vi "FCI_EON_Blob_Center.vi"(8 "error in (no error)":errorcluster, 10 "Coord ROI":T1 {"Contours"."Type" items=["No Selection", "Point", "Line", "Rectangle", "Oval", "Polygon", "Freehand Region", "Annulus", "Unused2", "Unused3", "Broken Line", "Freehand Line", "Rotated Rectangle"]}, 11 "Image In":T2(plugin-control)) -> (0 "error out":errorcluster, 1 "EON Area":dbl, 2 "EON Presence/Absence":bool, 3 "Blob Center":cluster{"Center X":dbl, "Center Y":dbl})   [LabVIEW 2019, in "Algorithm.lvclass"]
uses:
  FrameworkOverrides/Algorithm.lvclass
  <vilib>/vision/NI_Vision_Development_Module.lvlib
panel:
  out "Y Coord":dbl[](array[numeric])
  out "Number of Particles":i32
  out "subarray 2":dbl[](array[numeric])
  out "index of element":i32
  out "Array":bool[](array[boolean])
  out "X Coord":dbl[](array[numeric])
  out "Image 2":T2(plugin-control)
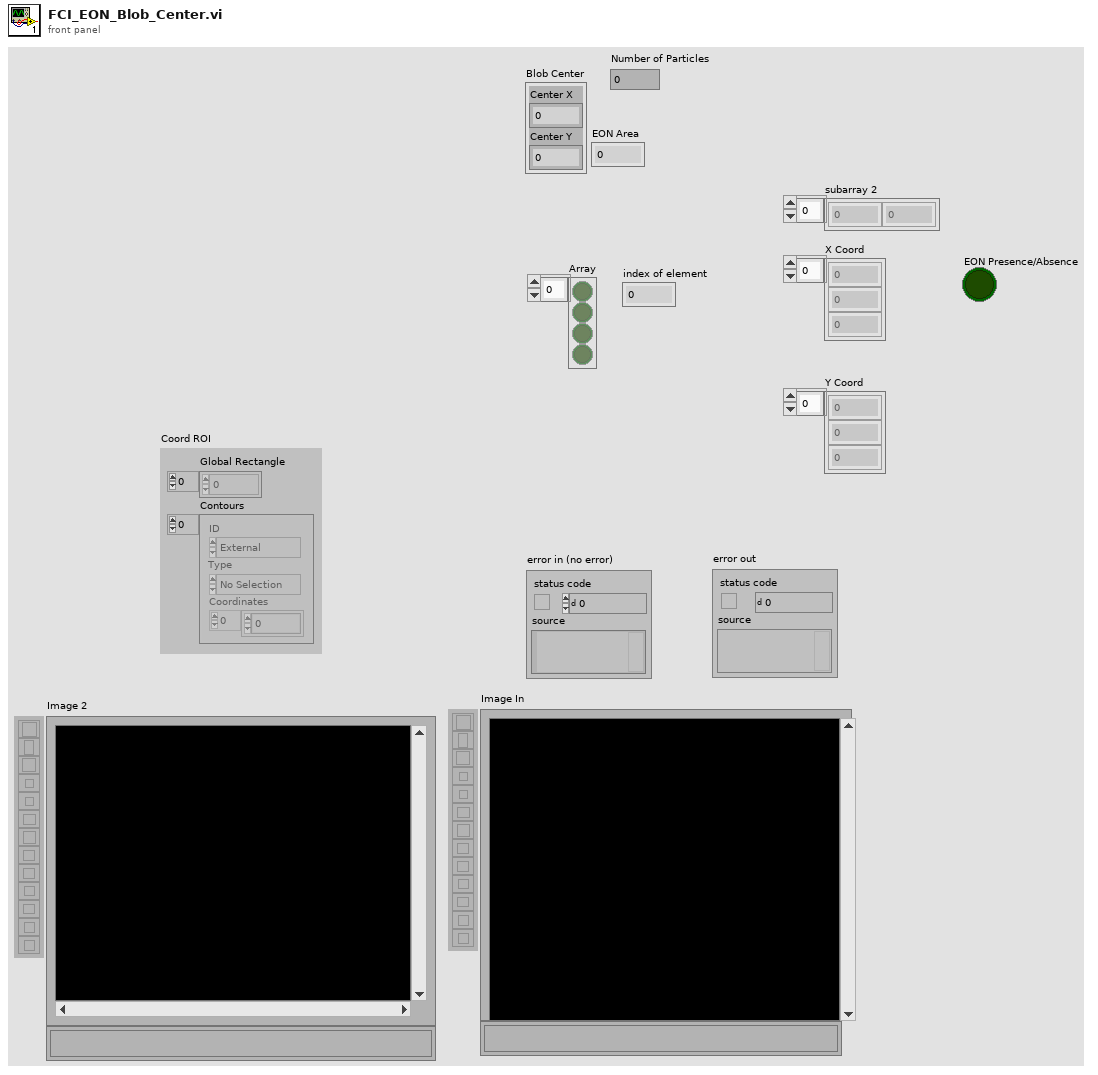
[diagram p1: front panel]
types:
  T1 = typedef "ROI Descriptor" = cluster{"Global Rectangle":i32[], "Contours":cluster{"ID":enum32{"External", "Internal"}, "Type":u32, "Coordinates":i32[]}[]}
  T2 = typedef "IMAQ Image.ctl" = refnum<image>
  T3 = typedef "Particle Parameters" = i32
  T4 = cluster{"Measurement Parameter":T3, "Range Lower Value":dbl, "Range Upper Value":dbl, "Range":bool, "Measurement Type":bool}[]
  T5 = typedef "Image Type" = u32
  T6 = typedef "IMAQ Rectangle" = cluster{"Left":i32, "Top":i32, "Right":i32, "Bottom":i32, "Rotation":dbl}
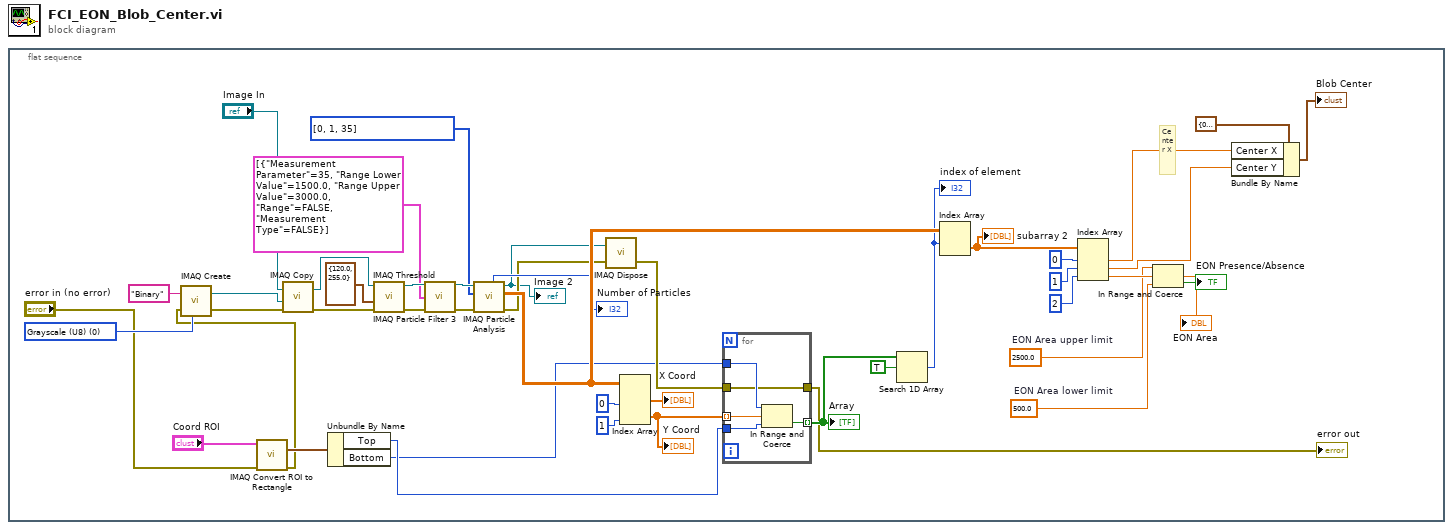
[diagram p0: block diagram]
diagram:
  n1 = flat-sequence {
    frame #0 {
      w18 = 500.0  # EON Area lower limit
      w19 = 2500.0  # EON Area upper limit
      w38 = T3[] [0, 1, 35] items=["Center of Mass X", "Center of Mass Y", "First Pixel X", "First Pixel Y", "Bounding Rect Left", "Bounding Rect Top", "Bounding Rect Right", "Bounding Rect Bottom", "Max Feret Diameter Start X", "Max Feret Diameter Start Y", "Max Feret Diameter End X", "Max Feret Diameter End Y", "Max Horiz. Segment Length Left", "Max Horiz. Segment Length Right", "Max Horiz. Segment Length Row", "-", "Bounding Rect Width", "Bounding Rect Height", "Bounding Rect Diagonal", "Perimeter", "Convex Hull Perimeter", "Holes' Perimeter", "Max Feret Diameter", "Equivalent Ellipse Major Axis", "Equivalent Ellipse Minor Axis", "Equivalent Ellipse Minor Axis (Feret)", "Equivalent Rect Long Side", "Equivalent Rect Short Side", "Equivalent Rect Diagonal", "Equivalent Rect Short Side (Feret)", "Average Horiz. Segment Length", "Average Vert. Segment Length", "Hydraulic Radius", "Waddel Disk Diameter", "-", "Area", "Holes' Area", "Particle & Holes' Area", "Convex Hull Area", "Image Area", "-", "Number of Holes", "Number of Horiz. Segments", "Number of Vert. Segments", "-", "Orientation", "Max Feret Diameter Orientation", "-", "% Area/Image Area", "% Area/(Particle & Holes' Area)", "Ratio of Equivalent Ellipse Axes", "Ratio of Equivalent Rect Sides", "-", "Elongation Factor", "Compactness Factor", "Heywood Circularity Factor", "Type Factor", "-", "Sum X", "Sum Y", "Sum XX", "Sum XY", "Sum YY", "Sum XXX", "Sum XXY", "Sum XYY", "Sum YYY", "-", "Moment of Inertia XX", "Moment of Inertia XY", "Moment of Inertia YY", "Moment of Inertia XXX", "Moment of Inertia XXY", "Moment of Inertia XYY", "Moment of Inertia YYY", "Norm. Moment of Inertia XX", "Norm. Moment of Inertia XY", "Norm. Moment of Inertia YY", "Norm. Moment of Inertia XXX", "Norm. Moment of Inertia XXY", "Norm. Moment of Inertia XYY", "Norm. Moment of Inertia YYY", "Hu Moment 1", "Hu Moment 2", "Hu Moment 3", "Hu Moment 4", "Hu Moment 5", "Hu Moment 6", "Hu Moment 7"] ("Pixel Measurements")
      w44 = T5 0 items=["Grayscale (U8)", "Grayscale (I16)", "Grayscale (SGL)", "Complex (CSG)", "RGB (U32)", "HSL (U32)", "RGB (U64)", "Grayscale (U16)"] ("Image Type")
      # "Center X"
      n2 = call "IMAQ Convert ROI to Rectangle"("error in (no error)"="error in (no error)", "ROI Descriptor"="Coord ROI") -> ("error out"=w4:errorcluster, "Rectangle"=w7:T6)  [unwired: 7 in]
      n3 = call "IMAQ Create"("Image Name"="Binary", "Image Type"=w44, "error in (no error)"=w4) -> ("New Image"=w43:T2, "error out"=w16:errorcluster)  [unwired: 2 in]
      n4 = call "IMAQ Copy"("error in (no error)"=w16, "Image Dst"=w43, "Image Src"="Image In") -> ("error out"=w22:errorcluster, "Image Dst Out"=w37:T2)  [unwired: 3 in]
      n5 = Unbundle By Name(w7) -> ("Top"=w3:i32, "Bottom"=w2:i32)
      n6 = call "IMAQ Threshold"("error in (no error)"=w22, "Range"=cluster{"Lower value":sgl, "Upper value":sgl} {"Lower value"=120.0, "Upper value"=255.0}, "Image Src"=w37) -> ("error out"=w42:errorcluster, "Image Dst Out"=w41:T2)  [unwired: 7 in]
      n7 = call "IMAQ Particle Filter 3"("Image Src"=w41, "Selection Values"=T4 [{"Measurement Parameter"=35, "Range Lower Value"=1500.0, "Range Upper Value"=3000.0, "Range"=FALSE, "Measurement Type"=FALSE}], "error in (no error)"=w42) -> ("Image Dst Out"=w40:T2, "error out"=w39:errorcluster)  [unwired: 10 in, 1 out]
      n8 = call "IMAQ Particle Analysis"("error in (no error)"=w39, "Pixel Measurements"=w38, "Image"=w40) -> ("error out"=w11:errorcluster, "Particle Measurements (Pixels)"=w33:dbl[][], "Image Out (duplicate)"=w10:T2, "Number of Particles"=→"Number of Particles":i32)  [unwired: 3 in, 2 out]
      "Image 2" <- w10
      n9 = call "IMAQ Dispose"("Image"=w10, "error in (no error)"=w11) -> ("error out"=w9:errorcluster)  [unwired: 4 in]
      n10 = Index Array(array=w33, index (col) #1=0 ("disabled index (col)"), index (col) #2=1 ("index (col)")) -> (element #1=→"X Coord":dbl[], element #2=w25:dbl[])  [unwired: 2 in]
      "Y Coord" <- w25
      n11 = for {
        tunnel: w25 -> [w50] mode=indexing
        tunnel: [w49] -> w35 mode=indexing
        tunnel: w2 -> [w48]
        tunnel: w3 -> [w47]
        tunnel: w9 -> [w46]
        tunnel: [w46] -> w8
        n12 = In Range and Coerce(upper limit=w48, x=w50, lower limit=w47) -> (In Range?=w49:bool)  [unwired: 1 out]
      }
      "Array" <- w35
      "error out" <- w8
      n13 = Search 1D Array(1D array=w35, element=TRUE) -> (index of element=w32:i32)  [unwired: 1 in]
      "index of element" <- w32
      n14 = Index Array(array=w33, index (row)=w32) -> (element=w31:dbl[])  [unwired: 1 in]
      "subarray 2" <- w31
      n15 = Index Array(array=w31, index #1=0 ("index"), index #2=1 ("index"), index #3=2 ("index")) -> (element #1=w14:dbl, element #2=w13:dbl, element #3=w20:dbl)
      "EON Area" <- w20
      n16 = In Range and Coerce(upper limit=w19, x=w20, lower limit=w18) -> (In Range?=→"EON Presence/Absence":bool)  [unwired: 1 out]
      n17 = Bundle By Name(cluster=cluster{"Center X":dbl, "Center Y":dbl} {"Center X"=0.0, "Center Y"=0.0} ("Cluster"), "Center X"=w14, "Center Y"=w13) -> (→"Blob Center":cluster{"Center X":dbl, "Center Y":dbl})
    }
  }
